vi "Sensor Locate.vi"   [LabVIEW 2020]
uses:
  Classes/Workspace/Pick Up Tool Area/Pick Up Tool Fixture.lvclass
  Drivers/Aerotech A3200/Motion/FreerunSingle.vi
  Classes/Controller/I-O/I-O.lvclass
  Classes/Routine/Pick and Place/Pick and Place.lvclass
  Classes/Controller/Motion/Motion.lvclass
  Classes/Controller/Controller.lvclass
types:
  T1 = typedef "Controller.lvclass/Controllers.ctl" = cluster{"I-O.lvclass":refnum<class "I-O.lvclass">, "Dispenser.lvclass":refnum<class "Dispenser.lvclass">, "Gantry":refnum<k24>}
  T2 = typedef "Fixture.lvclass/Workspace.ctl" = cluster{"XYZTheta":dbl[], "Workspace Valve":i32, "Workspace Sensor":i32}
  T3 = typedef "I-O.lvclass/Pin Map.ctl" = cluster{"Region Valves":i32[], "Extra Valves":dbl[][][], "Tool Primary Valve":i32, "Tool Secondary Valve":i32, "Region Sensors":i32[], "Extra Sensors":dbl[][][], "Tool Primary Sensor":dbl, "Tool Secondary Sensor":dbl, "Compression Sensor":dbl, "5V":i32}
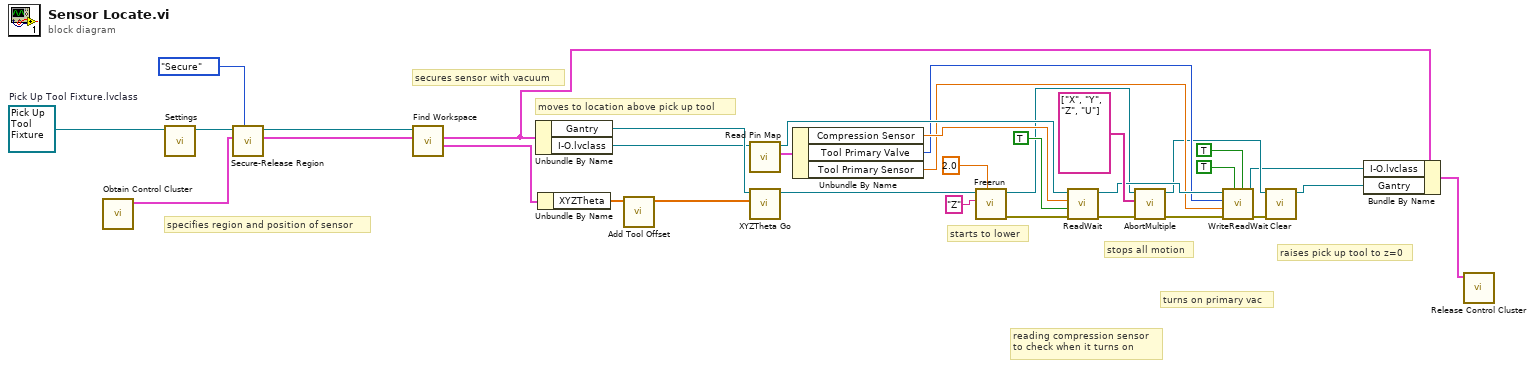
[diagram p0: block diagram]
diagram:
  w26 = refnum<class "Pick Up Tool Fixture.lvclass"> refnum  # Pick Up Tool Fixture.lvclass
  # "raises pick up tool to z=0"
  # "turns on primary vac"
  # "stops all motion"
  # "reading compression sensor\nto check when it turns on"
  # "starts to lower"
  # "moves to location above pick up tool"
  # "secures sensor with vacuum"
  # "specifies region and position of sensor"
  n1 = call "Obtain Control Cluster.vi"() -> ("Control Out"=w28:T1)  [unwired: 11 in]
  n2 = call-dynamic "Settings.vi"("Workspace in"=w26) -> ("Workspace out"=w34:refnum<class "Pick Up Tool Fixture.lvclass">)  [unwired: 9 in, 1 out]
  n3 = call-dynamic "Secure-Release Region.vi"("Action"=enum16{"Secure", "Release"}."Secure", "Control In"=w28, "Fixture in"=w34) -> ("Control Out"=w27:T1, "Fixture out"=w32:refnum<class "Pick Up Tool Fixture.lvclass">)  [unwired: 6 in, 1 out]
  n4 = call-dynamic "Find Workspace.vi"("Control In"=w27, "Workspace In"=w32) -> ("Workspace Out"=w31:T2, "Control Out"=w4:T1)  [unwired: 6 in, 2 out]
  n5 = Unbundle By Name(w4) -> ("Gantry"=w29:refnum<k24>, "I-O.lvclass"=w21:refnum<class "I-O.lvclass">)
  n6 = Unbundle By Name(w31) -> ("XYZTheta"=w30:dbl[])
  n7 = call "Add Tool Offset.vi"("XYZTheta"=w30) -> ("Array"=w25:dbl[])  [unwired: 10 in]
  n8 = call-dynamic "Read Pin Map.vi"("I-O in"=w21) -> ("Pin Map 2"=w20:T3, "I-O out"=w14:refnum<class "I-O.lvclass">)  [unwired: 8 in, 1 out]
  n9 = call "XYZTheta Go.vi"("XYZTheta In"=w25, "Gantry 2"=w29) -> ("Gantry 3"=w24:refnum<k24>)  [unwired: 7 in, 2 out]
  n10 = Unbundle By Name(w20) -> ("Compression Sensor"=w19:dbl, "Tool Primary Valve"=w12:i32, "Tool Primary Sensor"=w11:dbl)
  n11 = call-poly "Freerun.vi"("speed"=2.0, "axis name"="Z", "controller in"=w24) -> ("error out"=w17:errorcluster, "controller out"=w6:refnum<k24>)  [unwired: 7 in]
  n12 = call "ReadWait.vi"("error in (no error)"=w17, "Value"=TRUE, "Read"=w19, "I-O in"=w14) -> ("error out"=w16:errorcluster, "I-O out"=w13:refnum<class "I-O.lvclass">)  [unwired: 6 in]
  n13 = call "AbortMultiple.vi"("error in (no error)"=w16, "axis names"=string[] ["X", "Y", "Z", "U"], "controller in"=w6) -> ("error out"=w8:errorcluster, "controller out"=w5:refnum<k24>)  [unwired: 7 in]
  n14 = call "WriteReadWait.vi"("Read Value"=TRUE, "Write Value"=TRUE, "error in (no error)"=w8, "Read"=w11, "Write"=w12, "I-O in"=w13) -> ("error out"=w7:errorcluster, "I-O out"=w3:refnum<class "I-O.lvclass">)  [unwired: 4 in]
  n15 = call "Clear.vi"("error in (no error)"=w7, "Gantry 2"=w5) -> ("Gantry 3"=w2:refnum<k24>)  [unwired: 8 in, 1 out]
  n16 = Bundle By Name(cluster=w4, "I-O.lvclass"=w3, "Gantry"=w2) -> (w1:T1)
  n17 = call "Release Control Cluster.vi"("output cluster"=w1) -> ()  [unwired: 11 in]
